vi "Output Protection Status.vi"(8 "error in (no error)":errorcluster, 10 "Channel (1: Channel 1)":i32(ring)=1 items=["Channel 1"=1, "Channel 2"=2], 11 "VISA resource name":refnum<visa-resource-name>) -> (0 "error out":errorcluster, 1 "OCP Tripped?":bool, 2 "OVP Tripped?":bool, 3 "VISA resource name out":refnum<visa-resource-name>)   [LabVIEW 2013, in "Template - DC Power.lvlib"]
doc: "Returns over voltage protection (OVP) and over current protection (OCP) status for a desired channel."
uses:
  <instrlib>/_Template - DC Power/Template - DC Power.lvlib
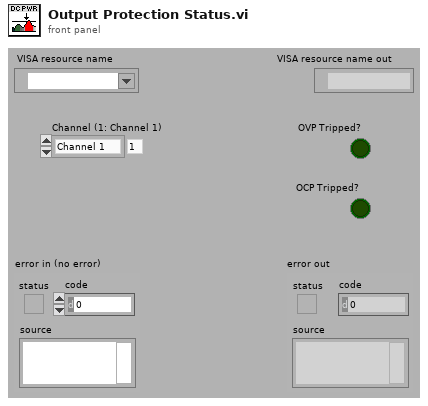
[diagram p1: front panel]
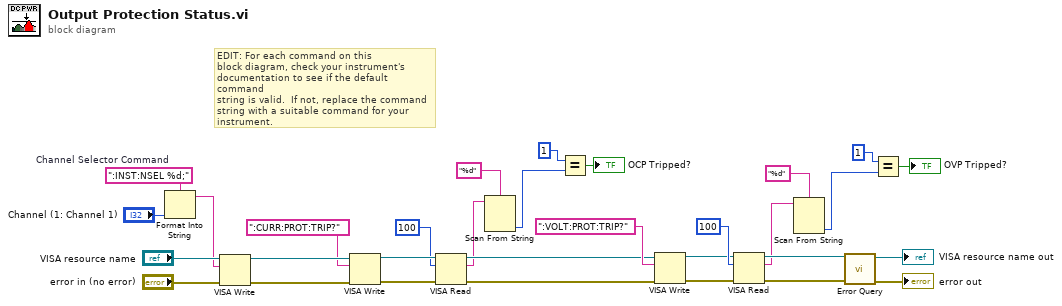
[diagram p0: block diagram]
diagram:
  w27 = ":INST:NSEL %d;"  # Channel Selector Command
  # "EDIT: For each command on this\nblock diagram, check your instrument's\ndocumentation to see if the default command\nstring is valid.  If not, replace the command\nstring with a suitable command for your\ninstrument."
  n1 = Format Into String(format string=w27, "Channel (1: Channel 1)") -> (resulting string=w25:string)  [unwired: 2 in, 1 out]
  n2 = VISA Write(VISA resource name="VISA resource name", write buffer=w25, error in (no error)="error in (no error)") -> (VISA resource name out=w24:refnum<visa-resource-name>, error out=w23:errorcluster)  [unwired: 1 out]
  n3 = VISA Write(VISA resource name=w24, write buffer=":CURR:PROT:TRIP?", error in (no error)=w23) -> (VISA resource name out=w20:refnum<visa-resource-name>, error out=w21:errorcluster)  [unwired: 1 out]
  n4 = VISA Read(VISA resource name=w20, byte count=u32 100, error in (no error)=w21) -> (VISA resource name out=w12:refnum<visa-resource-name>, read buffer=w8:string, error out=w11:errorcluster)  [unwired: 1 out]
  n5 = Scan From String(format string="%d", input string=w8) -> (output 1=w2:i32)  [unwired: 3 in, 3 out]
  n6 = Equal?(x=1, y=w2) -> (x = y?=→"OCP Tripped?":bool)
  n7 = VISA Write(VISA resource name=w12, write buffer=":VOLT:PROT:TRIP?", error in (no error)=w11) -> (VISA resource name out=w16:refnum<visa-resource-name>, error out=w15:errorcluster)  [unwired: 1 out]
  n8 = VISA Read(VISA resource name=w16, byte count=u32 100, error in (no error)=w15) -> (VISA resource name out=w10:refnum<visa-resource-name>, read buffer=w4:string, error out=w9:errorcluster)  [unwired: 1 out]
  n9 = Scan From String(format string="%d", input string=w4) -> (output 1=w1:i32)  [unwired: 3 in, 3 out]
  n10 = call <instrlib>:"Error Query.vi"("error in (no error)"=w9, "VISA resource name"=w10) -> ("error out"=→"error out":errorcluster, "VISA resource name out"=→"VISA resource name out":refnum<visa-resource-name>)  [unwired: 6 in, 2 out]
  n11 = Equal?(x=1, y=w1) -> (x = y?=→"OVP Tripped?":bool)
